vi "Clear Data3.vi"(0 "Data In":T2, 2 "Time":u32, 3 "error in (no error)":errorcluster) -> (7 "Data Out":T2, 8 "Timeout":bool, 9 "State":T1=enum."Initialize", 10 "error out":errorcluster)   [LabVIEW 2014]
uses:
  controls/Data1.ctl
  controls/Payjson.ctl
  controls/State.ctl
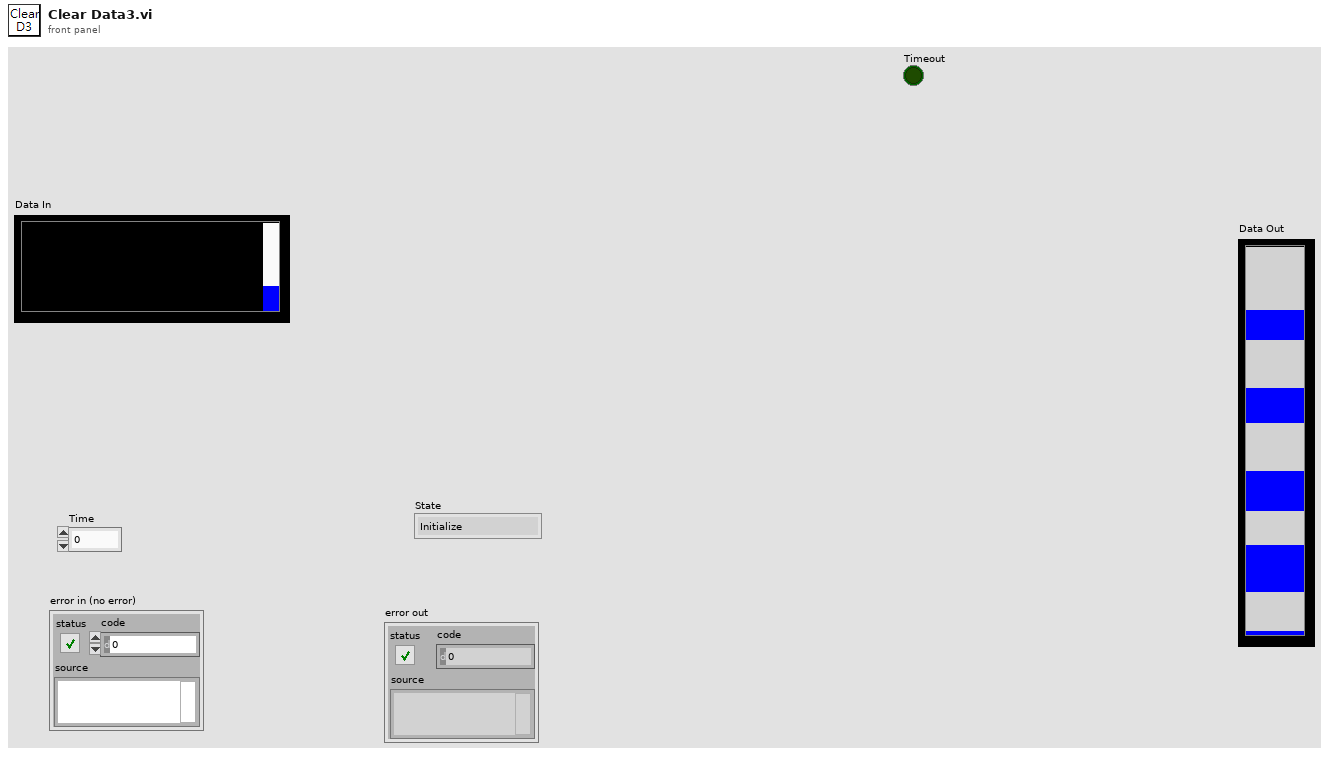
[diagram p1: front panel]
types:
  T1 = typedef "State.ctl" = enum16{"int", "Initalize0", "Initialize", "Wait for Scan", "State 1", "State 2", "NG", "NG1", "OK", "OKNG", "OKNG1", "Exit"}
  T2 = typedef "Data1.ctl" = cluster{"Date":string, "BarCode1":string, "BarCode2":string, "BarCode3":string, "Message":string, "OK Count":u16, "NG Count":u16, "Total Count":u16, "ModelData":string[][], "OK&NG":bool, "COM1":refnum<visa-resource-name>, "COM2":refnum<visa-resource-name>, "IO":i32, "Time":u32, "TCP":refnum<k5>, "TCP 2":refnum<k5>, "COM1 2":refnum<visa-resource-name>, "CheckNum":string, "BarCode1_1":string, "BarCode2_1":string, "BarCode3_1":string, "日期":string, "機種":string, "機號":string, "商品條碼1":string, "OK_1":string, "OK":string, "NG":string, "NG_1":string, "Total":string, "Total_1":string, "ClaerTime":u32, "Pjson":T3, "LotNo":string[], "CheckParsArray":string[], "BarCode4":string, "BarCode4_1":string, "商品條碼2":string, "BarCode5":string, "BarCode5_1":string, "商品條碼3":string, "ReScanNG":i32, "NGTimeCT":u32}
  T3 = typedef "Payjson.ctl" = cluster{"DEPT":string, "LINE":string, "STANO":string, "WORKNO":string, "PRODSN":string, "COMPNTID":string, "COMPNTLOT":string, "COMPNTSN":string, "USEDQTY":i16, "OPDATE":string, "OPUSER":string, "RECVDATE":string, "MMODU":string}[]
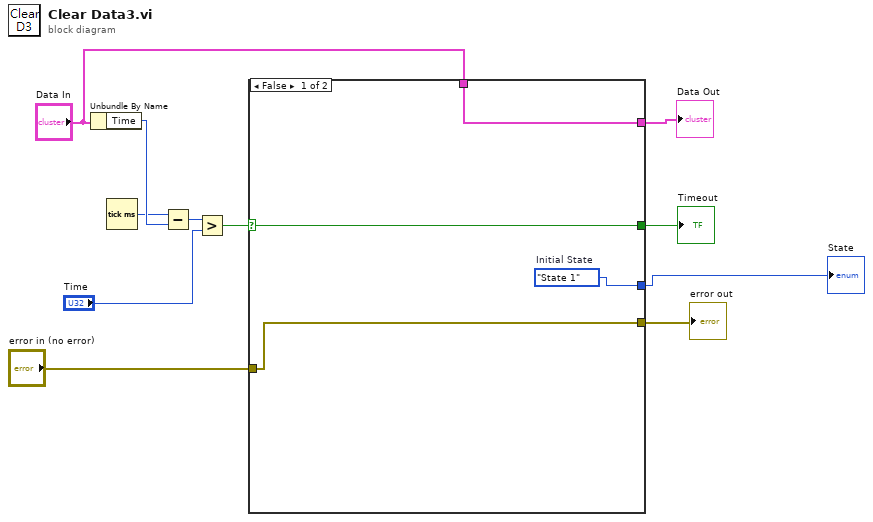
[diagram p0: block diagram]
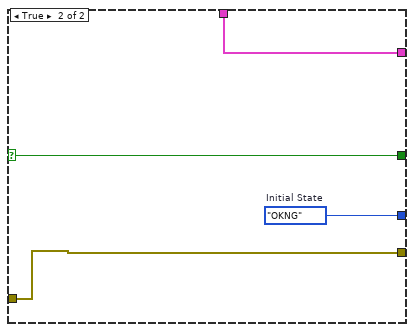
[diagram p2: hidden frame]
diagram:
  n1 = Unbundle By Name("Data In") -> ("Time"=w11:u32)
  n2 = Tick Count (ms)() -> (millisecond timer value=w10:u32)
  n3 = Subtract(x=w10, y=w11) -> (x-y=w9:u32)
  n4 = Greater?(x=w9, y="Time") -> (0:w7:bool)
  n5 = case shown="False" w7 {
    selector: w7 -> [w13 w17]
    tunnel: "Data In" -> [w15 w18]
    tunnel: [w15 w18] -> w5
    tunnel: "error in (no error)" -> [w14 w19]
    tunnel: [w14 w19] -> w3
    tunnel: [w13 w17] -> w2
    tunnel: [w12 w16] -> w1
    frame False {
      w12 = State."State 1"  # Initial State
    }
    frame True {
      w16 = State."OKNG"  # Initial State
    }
  }
  "Data Out" <- w5
  "error out" <- w3
  "Timeout" <- w2
  "State" <- w1
